vi "ReadMatlabLogFiles_v1.vi"(5 "use system decimal point (T)":bool, 9 "FileName":string="LogFile", 11 "sequence list REF":refnum<vi>) -> (0 "error out":errorcluster, 1 "sequence cluster":T1, 2 "sequence NbX NbZ":dbl[][](array[numeric]), 3 "logfile":string[][](array[string]), 4 "Phase array unit":dbl[](array[numeric]), 6 "all values":dbl[][](array[numeric]))   [LabVIEW 2018, in "RW_Protocols.lvlib"]
uses:
  RW_Protocols.lvlib
  FileType.ctl
  <vilib>/Utility/file.llb/Read Delimited Spreadsheet (string).vi
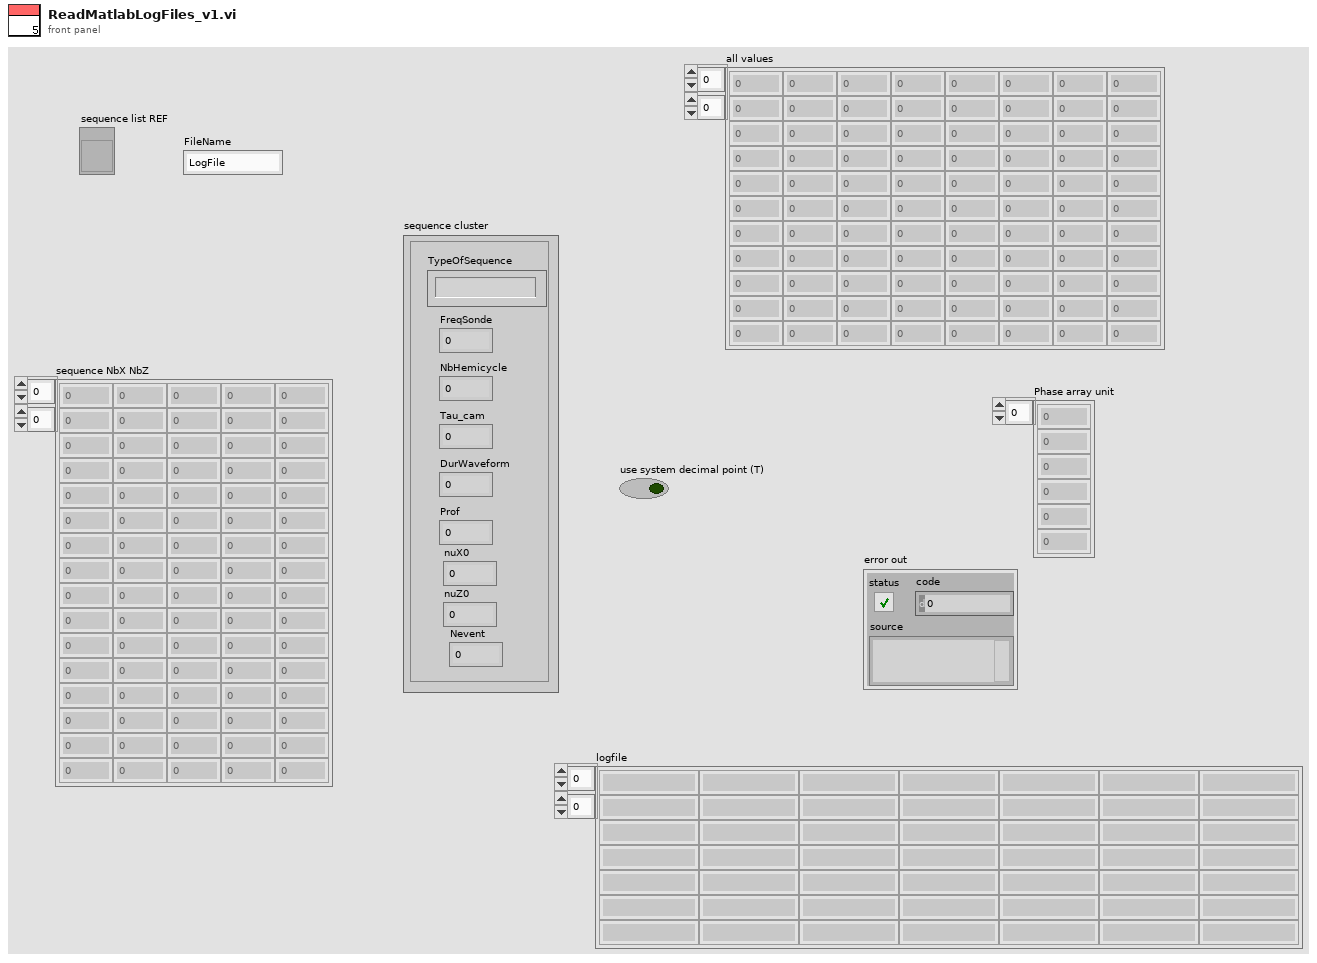
[diagram p1: front panel]
types:
  T1 = cluster{"TypeOfSequence":string, "FreqSonde":dbl, "NbHemicycle":dbl, "Tau_cam":dbl, "DurWaveform":dbl, "Prof":dbl, "Nevent":i32, "nuX0":dbl, "nuZ0":dbl}
  T2 = typedef "RW_Protocols.lvlib/FileType.ctl" = enum16{"png", "csv", "tiff", "dat", "bin", "txt"}
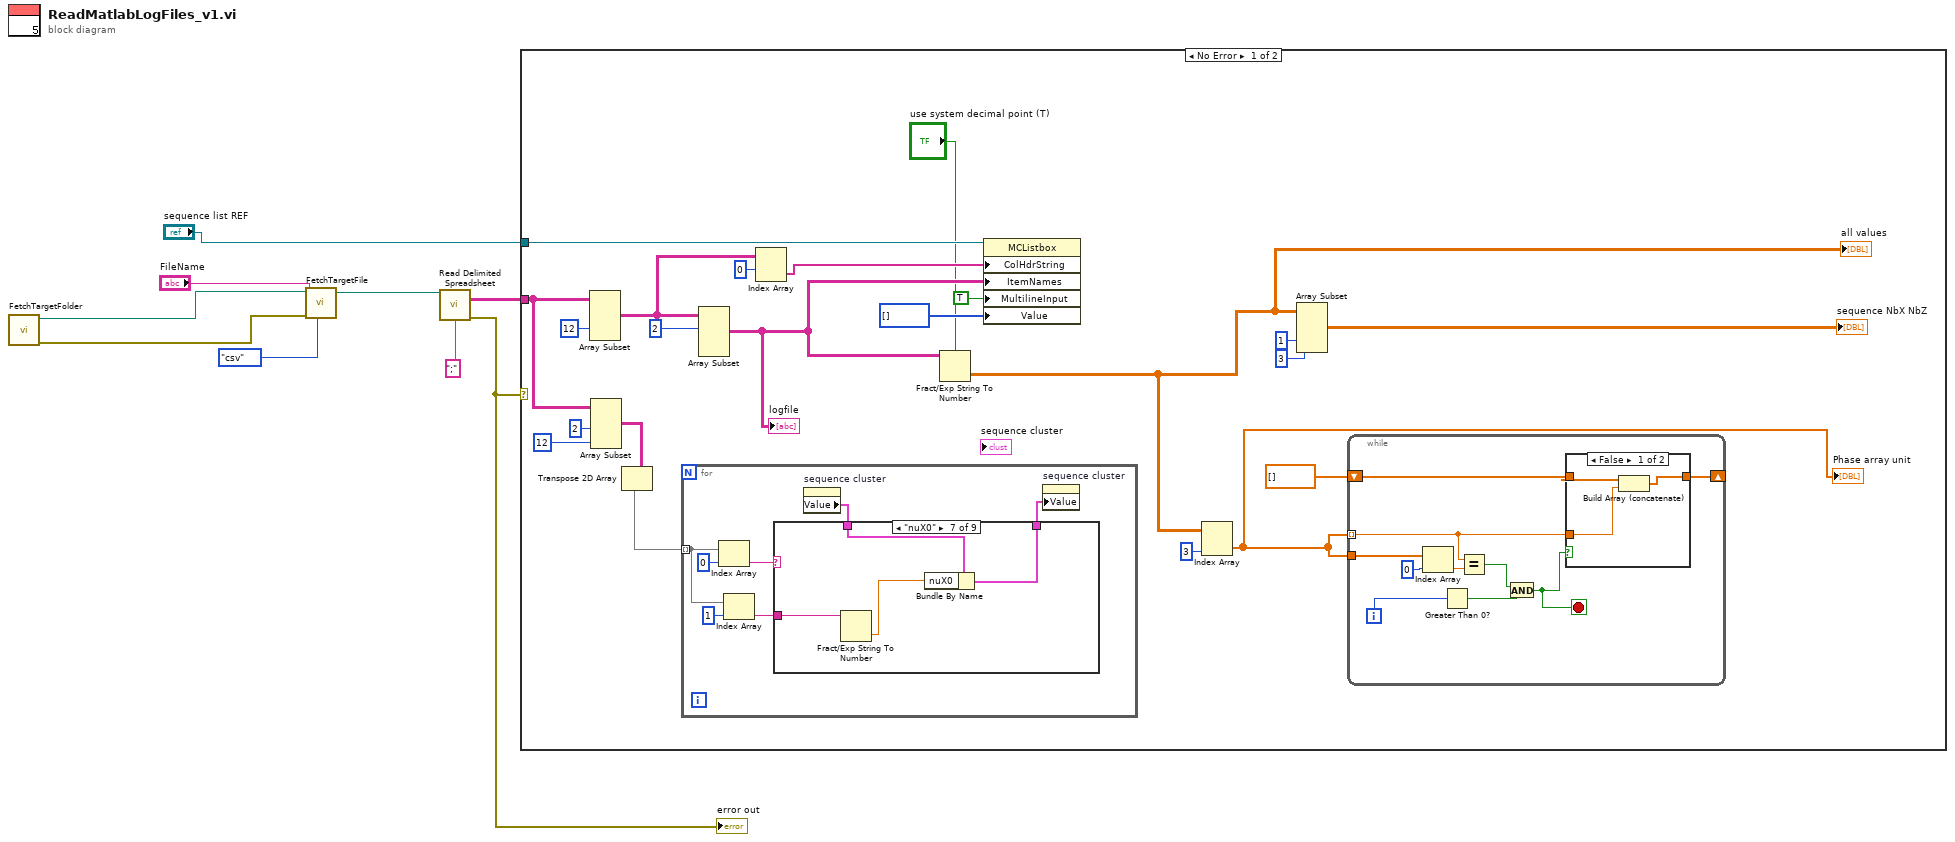
[diagram p0: block diagram]
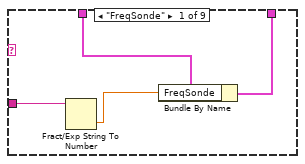
[diagram p3: hidden frame]
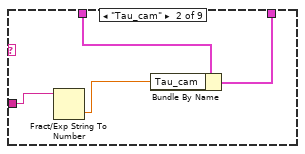
[diagram p4: hidden frame]
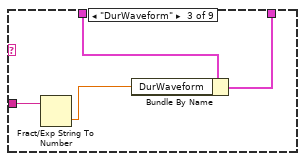
[diagram p5: hidden frame]
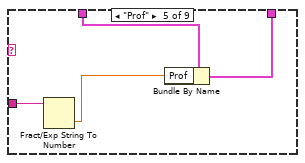
[diagram p7: hidden frame]
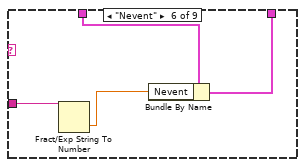
[diagram p8: hidden frame]
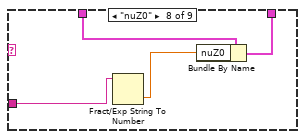
[diagram p9: hidden frame]
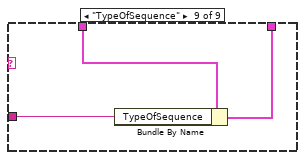
[diagram p10: hidden frame]
diagram:
  n1 = call "FetchTargetFolder.vi"() -> ("error out"=w1:errorcluster, "Full File Path"=w2:path)  [unwired: 10 in]
  n2 = call "FetchTargetFile.vi"("file type"=FileType."csv", "error in (no error)"=w1, "FileName"="FileName", "Target Folder"=w2) -> ("Full File Path"=w7:path)  [unwired: 6 in, 1 out]
  n3 = call-poly <vilib>:"Read Delimited Spreadsheet.vi"("file path (dialog if empty)"=w7, "delimiter (\\t)"=";" ("delimiter (\\t)")) -> ("all rows"=w5:string[][], "error out"=w4:errorcluster)  [unwired: 8 in, 4 out]
  "error out" <- w4
  n4 = case shown="No Error" w4 {
    tunnel: "sequence list REF" -> [w27 _]
    tunnel: w5 -> [w19 _]
    frame No Error {
      n5 = Array Subset(array=w19, index (col)=12 ("index")) -> (w28:string[][])  [unwired: 3 in]
      n6 = Array Subset(array=w19, length (row)=2 ("length"), length (col)=12 ("length")) -> (w20:string[][])  [unwired: 2 in]
      n7 = Transpose 2D Array(2D array=w20) -> (transposed array=w21:string[][])
      n8 = for {
        tunnel: w21 -> [w51] mode=indexing
        n9 = Index Array(array=w51, index=0) -> (element=w46:string)
        n10 = Index Array(array=w51, index=1) -> (element=w49:string)
        n11 = property on="sequence cluster" class="Clust (strict)"() -> ("Value"=w48:T1)  [unwired: 2 in, 2 out]
        n12 = case shown="\"nuX0\"" w46 {
          tunnel: w49 -> [w54 w58 w62 _ w67 w71 w75 w80 w84]
          tunnel: w48 -> [w56 w60 w63 w65 w69 w73 w77 w78 w83]
          tunnel: [w55 w59 w64 w65 w68 w72 w76 w79 w82] -> w47
          frame "FreqSonde" {
            n13 = Fract/Exp String To Number(string=w54) -> (number=w53:dbl)  [unwired: 3 in, 1 out]
            n14 = Bundle By Name(cluster=w56, "FreqSonde"=w53) -> (w55:T1)
          }
          frame "Tau_cam" {
            n15 = Fract/Exp String To Number(string=w58) -> (number=w57:dbl)  [unwired: 3 in, 1 out]
            n16 = Bundle By Name(cluster=w60, "Tau_cam"=w57) -> (w59:T1)
          }
          frame "DurWaveform" {
            n17 = Fract/Exp String To Number(string=w62) -> (number=w61:dbl)  [unwired: 3 in, 1 out]
            n18 = Bundle By Name(cluster=w63, "DurWaveform"=w61) -> (w64:T1)
          }
          frame Default {
          }
          frame "Prof" {
            n19 = Fract/Exp String To Number(string=w67) -> (number=w66:dbl)  [unwired: 3 in, 1 out]
            n20 = Bundle By Name(cluster=w69, "Prof"=w66) -> (w68:T1)
          }
          frame "Nevent" {
            n21 = Fract/Exp String To Number(string=w71) -> (number=w70:dbl)  [unwired: 3 in, 1 out]
            n22 = Bundle By Name(cluster=w73, "Nevent"=w70) -> (w72:T1)
          }
          frame "nuX0" {
            n23 = Fract/Exp String To Number(string=w75) -> (number=w74:dbl)  [unwired: 3 in, 1 out]
            n24 = Bundle By Name(cluster=w77, "nuX0"=w74) -> (w76:T1)
          }
          frame "nuZ0" {
            n25 = Fract/Exp String To Number(string=w80) -> (number=w81:dbl)  [unwired: 3 in, 1 out]
            n26 = Bundle By Name(cluster=w78, "nuZ0"=w81) -> (w79:T1)
          }
          frame "TypeOfSequence" {
            n27 = Bundle By Name(cluster=w83, "TypeOfSequence"=w84) -> (w82:T1)
          }
        }
        n28 = property on="sequence cluster" class="Clust (strict)"("Value"=w47) -> ()  [unwired: 2 in, 2 out]
      }
      n29 = Array Subset(array=w28, index (row)=2 ("index")) -> (w18:string[][])  [unwired: 3 in]
      "logfile" <- w18
      n30 = Index Array(array=w28, index (row)=0) -> (element=w26:string[])  [unwired: 1 in]
      n31 = Fract/Exp String To Number(use system decimal point (T)="use system decimal point (T)", string=w18) -> (number=w15:dbl[][])  [unwired: 2 in, 1 out]
      "all values" <- w15
      n32 = property class="MCListbox"(reference=w27, "ColHdrString"=w26, "ItemNames"=w18, "MultilineInput"=TRUE ("Multiple Line Input"), "Value"=i32[] []) -> ()  [unwired: 1 in, 2 out]
      n33 = Index Array(array=w15, index (col)=3 ("disabled index (col)")) -> (element=w10:dbl[])  [unwired: 1 in]
      "Phase array unit" <- w10
      n34 = Array Subset(array=w15, index (col)=1 ("index"), length (col)=3 ("length")) -> (→"sequence NbX NbZ":dbl[][])  [unwired: 2 in]
      n35 = while {
        shift-right: [w32] -> _
        shift-left: dbl[] [] -> [w37]
        tunnel: w10 -> [w33] mode=indexing
        tunnel: w10 -> [w35]
        i -> [w40]
        stop <- w36 stop-if-true
        n36 = Index Array(array=w35, index=0) -> (element=w34:dbl)
        n37 = Greater Than 0?(x=w40) -> (x > 0?=w39:bool)
        n38 = Equal?(x=w33, y=w34) -> (x = y?=w38:bool)
        n39 = And(x=w38, y=w39) -> (x .and. y?=w36:bool)
        n40 = case shown="False" w36 {
          tunnel: [w44 w45] -> w32
          tunnel: w37 -> [w43 w45]
          tunnel: w33 -> [w42 _]
          frame False {
            n41 = Build Array (concatenate)(w43, w42) -> (w44:dbl[])
          }
          frame True {
          }
        }
      }
    }
    frame Error {
    }
  }
